vi "Get Property.vi"(0 "video in":refnum<class "MSC Video.lvclass">, 1 "Camera Stream Property":T1=3 items=["Position msec", "Position frames", "Position avi ratio", "Frame Width", "Frame Height", "FPS", "FourCC codec", "Frame Count", "Format", "Mode", "Brightness", "Contrast", "Saturation", "Hue", "Gain", "Exposure", "Convert RGB", "White Balance U", "Rectification", "Monochrome", "Sharpness", "Auto Exposure", "Gamma", "Temperature", "Trigger", "Trigger Delay", "White Balance V", "Zoom", "Focus", "Guid", "ISO Speed", "Max DV1394", "Backlight", "Pan", "Tilt", "Rolls", "Iris", "Settings", "Buffersize"], 5 "error in (no error)":errorcluster) -> (14 "video out":refnum<class "MSC Video.lvclass">, 15 "propertyValue":dbl, 19 "error out":errorcluster)   [LabVIEW 2014, in "MSC Video.lvclass"]
doc: "Returns a selected Camera Stream Property."
uses:
  MSC Video.lvclass
  controls/Stream Property.ctl
  MSC Video.lvclass/MSC Video.ctl
  Dependencies/x86/MSC I Process32.dll
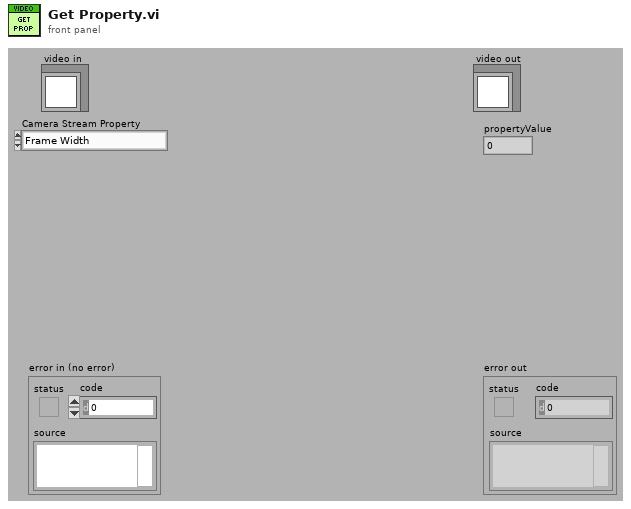
[diagram p1: front panel]
types:
  T1 = typedef "MSC Video.lvclass/Stream Property.ctl" = u16
  T2 = typedef "MSC Video.lvclass/Video.ctl" = cluster{"Pointer":u64, "CamID":i32, "File Path":path, "Network Address":string, "opened":bool}
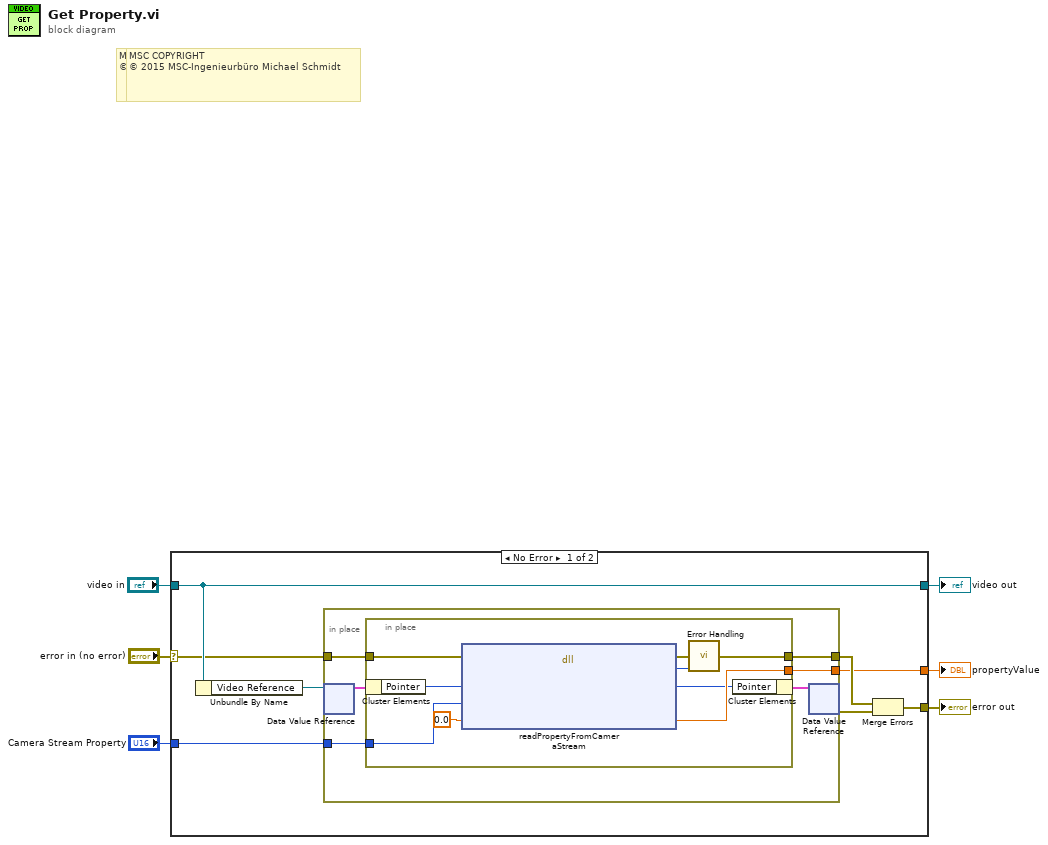
[diagram p0: block diagram]
diagram:
  # "MSC COPYRIGHT\n© 2016 MSC-Ingenieurbüro Michael Schmidt"
  # "MSC COPYRIGHT\n© 2016 MSC-Ingenieurbüro Michael Schmidt"
  # "MSC COPYRIGHT\n© 2015 MSC-Ingenieurbüro Michael Schmidt"
  n1 = case shown="No Error" "error in (no error)" {
    selector: "error in (no error)" -> [w8 w31]
    tunnel: [w7 w31] -> w5
    tunnel: [w14 w30] -> w3
    tunnel: "video in" -> [w14 w30]
    tunnel: "Camera Stream Property" -> [w10 _]
    tunnel: [w9 _] -> w1
    frame No Error {
      n2 = Unbundle By Name(w14) -> ("Video Reference"=w11:refnum<data-value>)
      n3 = in-place {
        in-place-border: w8 -> [w18]
        in-place-border: [w17] -> w12
        in-place-border: [w16] -> w9
        in-place-border: w10 -> [w15]
        n4 = in-place-dvr #1(w11) -> (w19:T2)  [unwired: 1 out]
        n5 = in-place {
          in-place-border: w18 -> [w22]
          in-place-border: [w29] -> w17
          in-place-border: [w24] -> w16
          in-place-border: w15 -> [w23]
          n6 = in-place-cluster #2(w19) -> ("Pointer"=w28:u64)
          n7 = dll-call lib="C:/Users/MSC/LabVIEW Projekte/LV 2014/MSC I-Process/user.lib/MSC-I Process/Dependencies/x86/MSC I Process*.dll" fn="readPropertyFromCameraStream"(error in=w22, "streamPointer"=w28, "propertyID"=w23, "propertyValue"=0.0) -> (error out=w27:errorcluster, "error"=w26:i32, "streamPointer"=w21:u64, "propertyValue"=w24:dbl)  [unwired: 3 in, 1 out]
          n8 = call "Error Handling.vi"("error in (no error)"=w27, "return type"=w26) -> ("error out"=w29:errorcluster)  [unwired: 12 in, 1 out]
          n9 = in-place-cluster #2("Pointer"=w21) -> (w20:T2)
        }
        n10 = in-place-dvr #1(w20) -> (w13:errorcluster)  [unwired: 1 out]
      }
      n11 = Merge Errors(w12, w13) -> (w7:errorcluster)
    }
    frame Error {
    }
  }
  "error out" <- w5
  "video out" <- w3
  "propertyValue" <- w1
